vi "Read Actual Sample Rate.vi"(8 "error in (no error)":errorcluster, 11 "Thermometer DAQmx Config in":refnum<class "Thermometer DAQmx Config.lvclass">) -> (0 "error out":errorcluster, 2 "Actual Sample Rate":dbl format="%#_g Hz", 3 "Thermometer DAQmx Config out":refnum<class "Thermometer DAQmx Config.lvclass">)   [LabVIEW 2023, in "Thermometer.lvlib" / "Thermometer DAQmx.lvlib" / "Thermometer DAQmx Config.lvclass"]
uses:
  Thermometer DAQmx Config.lvclass
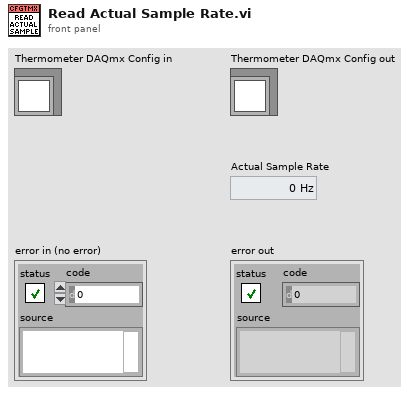
[diagram p1: front panel]
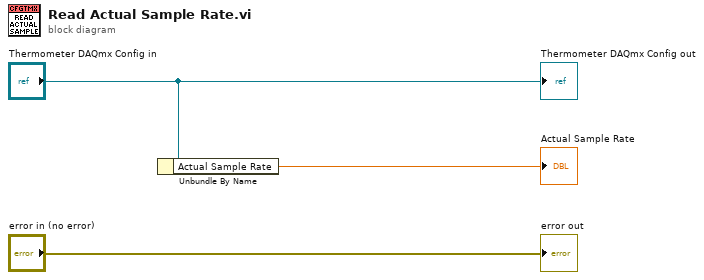
[diagram p0: block diagram]
diagram:
  n1 = Unbundle By Name("Thermometer DAQmx Config in") -> ("Actual Sample Rate"=→"Actual Sample Rate":dbl)
  "error out" <- "error in (no error)"
  "Thermometer DAQmx Config out" <- "Thermometer DAQmx Config in"
